vi "tankdataOLD.vi"(7 "LabVIEW Web Service Request":refnum<class "Web Request.lvclass">) -> ()   [LabVIEW 2019]
uses:
  <vilib>/wsapi/Web Request.lvclass
  Type Defs/JSON_Channel.ctl
  Type Defs/JSON_Pump.ctl
panel:
  # "Use the Web Service Request input terminal to call the VIs on the Web Services palette. Do not remove it from the connector pane unless you don't need access to the palette."
  # "Each additional control wired to the connector pane will be available as an input in the URL. To include an indicator in terminal-mode output (the default setting), it must also be wired to the connector pane."
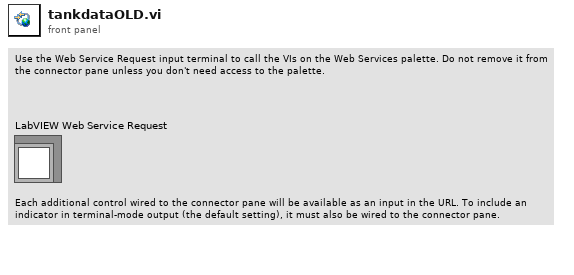
[diagram p1: front panel]
types:
  T1 = typedef "JSON_Tank.ctl" = cluster{"number":u16, "building":string, "room":string, "ipAddress":string, "profileName":string, "caNumber":string, "ctrlType":string, "mode":string, "channels":T2[], "pumps":T3[]}
  T2 = typedef "JSON_Channel.ctl" = cluster{"name":string, "tag":string, "data":string, "type":string, "unit":string}
  T3 = typedef "JSON_Pump.ctl" = cluster{"position":u8, "enabled":bool, "command":string, "channels":T2[], "elapsedTime":string}
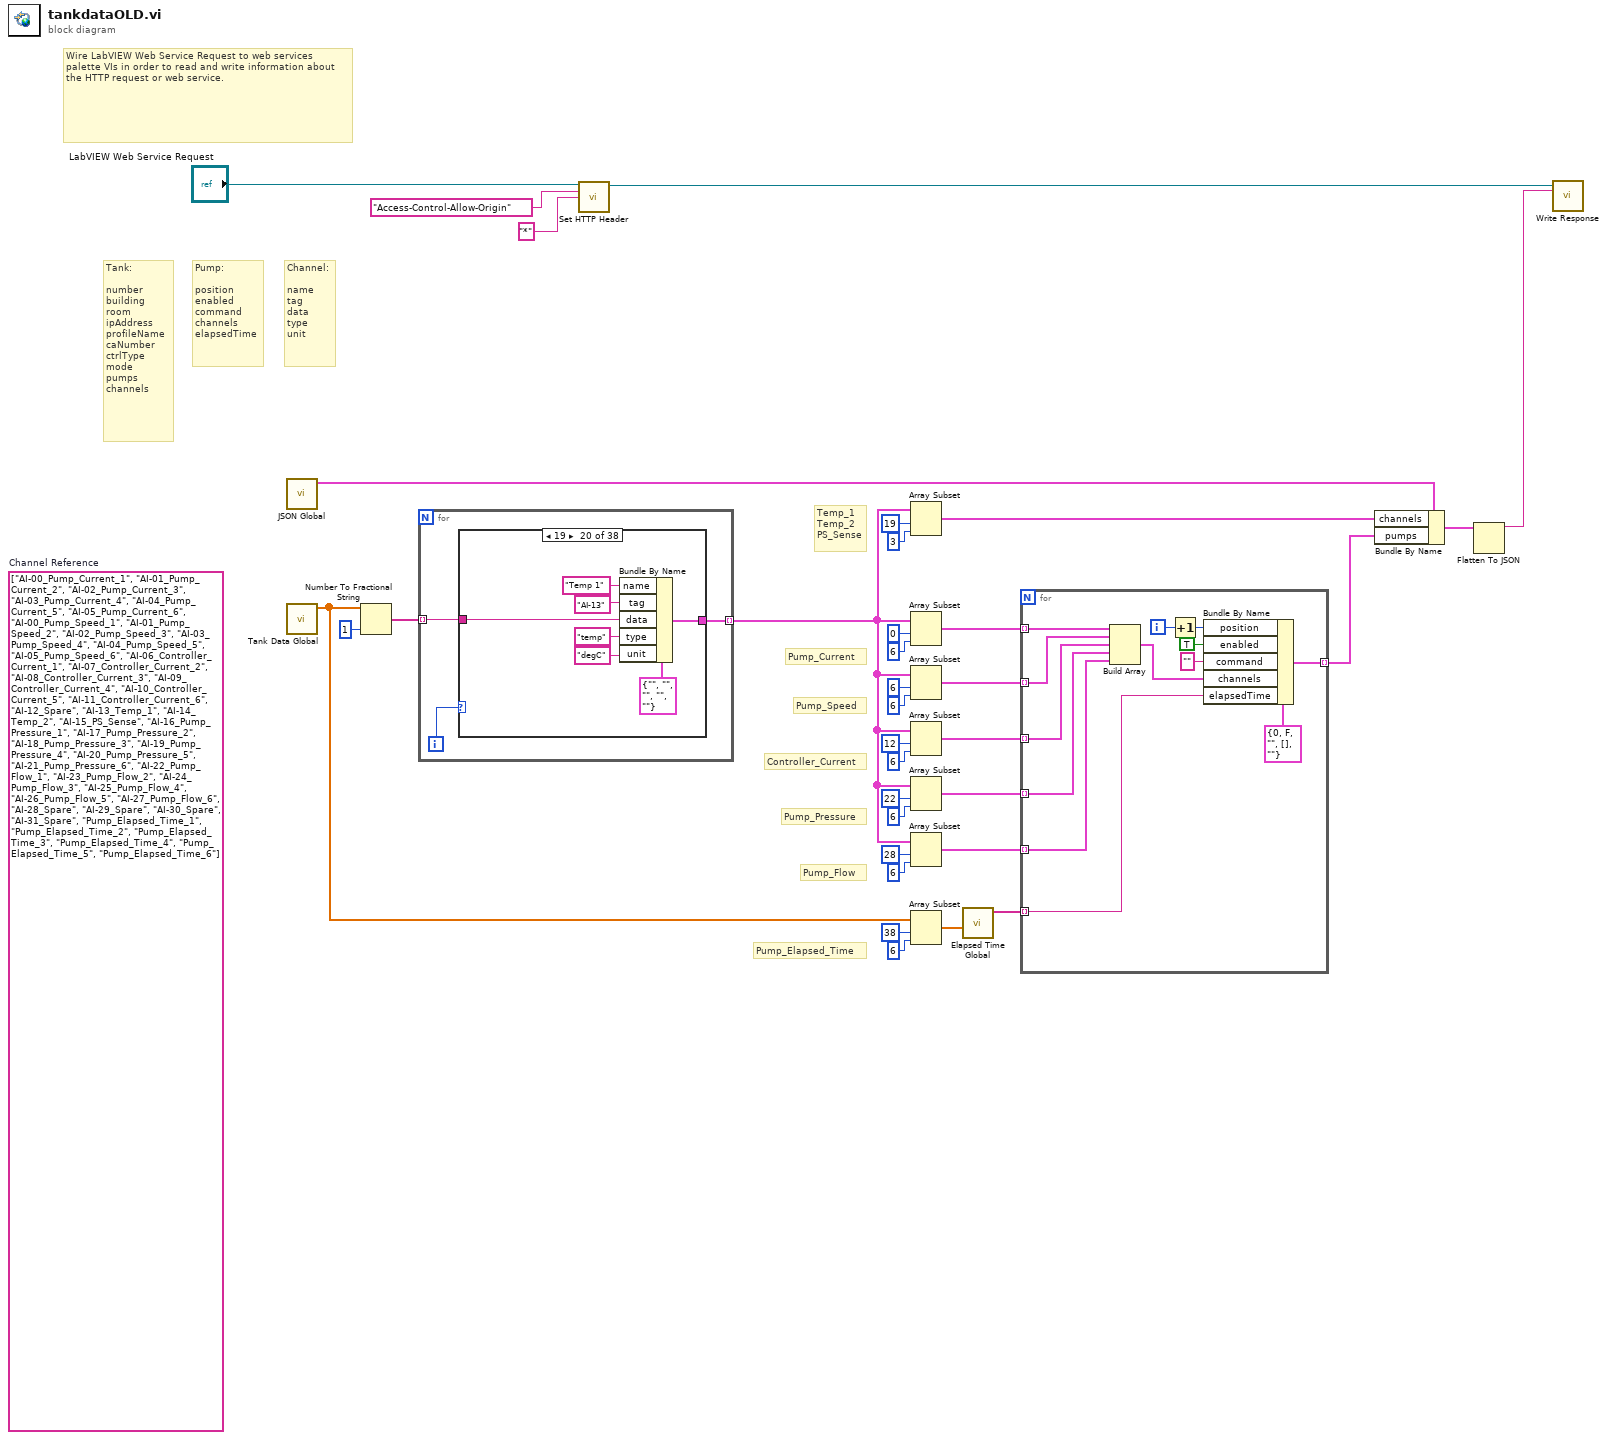
[diagram p0: block diagram]
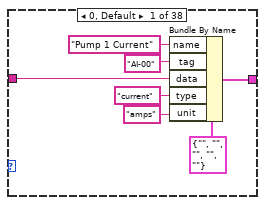
[diagram p2: hidden frame]
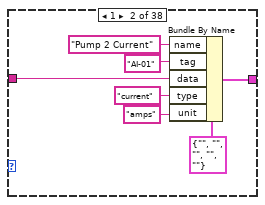
[diagram p3: hidden frame]
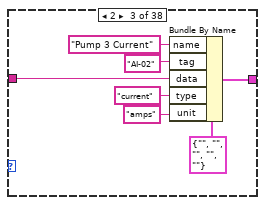
[diagram p4: hidden frame]
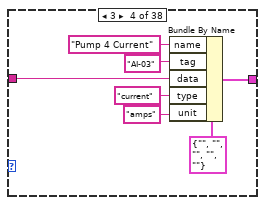
[diagram p5: hidden frame]
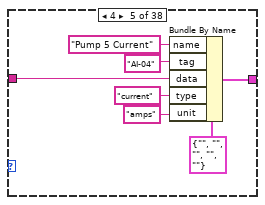
[diagram p6: hidden frame]
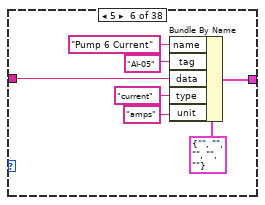
[diagram p7: hidden frame]
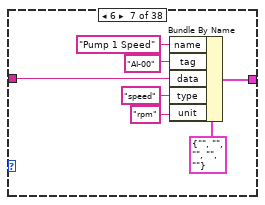
[diagram p8: hidden frame]
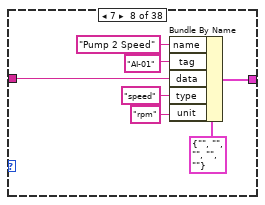
[diagram p9: hidden frame]
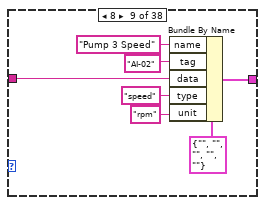
[diagram p10: hidden frame]
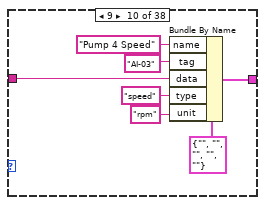
[diagram p11: hidden frame]
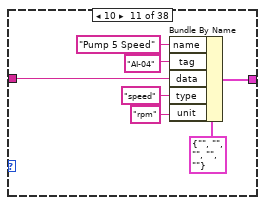
[diagram p12: hidden frame]
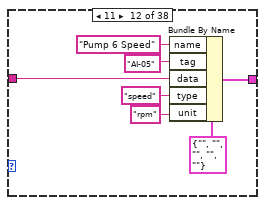
[diagram p13: hidden frame]
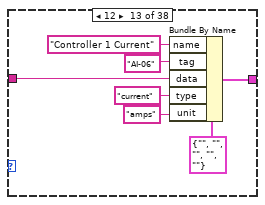
[diagram p14: hidden frame]
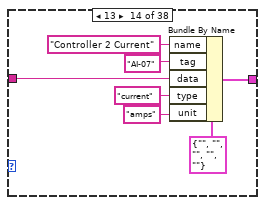
[diagram p15: hidden frame]
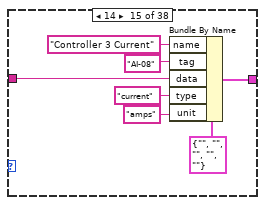
[diagram p16: hidden frame]
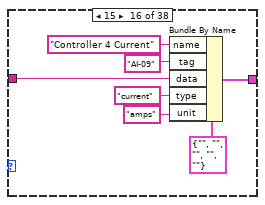
[diagram p17: hidden frame]
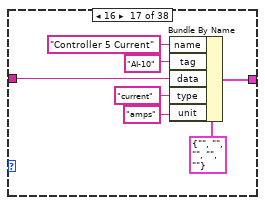
[diagram p18: hidden frame]
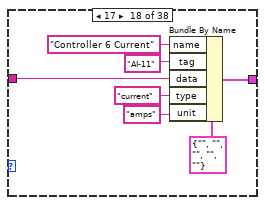
[diagram p19: hidden frame]
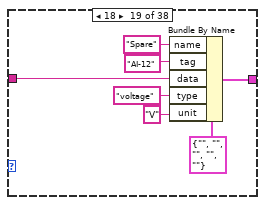
[diagram p20: hidden frame]
diagram:
  (unwired) string[] ["AI-00_Pump_Current_1", "AI-01_Pump_Current_2", "AI-02_Pump_Current_3", "AI-03_Pump_Current_4", "AI-04_Pump_Current_5", "AI-05_Pump_Current_6", "AI-00_Pump_Speed_1", "AI-01_Pump_Speed_2", "AI-02_Pump_Speed_3", "AI-03_Pump_Speed_4", "AI-04_Pump_Speed_5", "AI-05_Pump_Speed_6", "AI-06_Controller_Current_1", "AI-07_Controller_Current_2", "AI-08_Controller_Current_3", "AI-09_Controller_Current_4", "AI-10_Controller_Current_5", "AI-11_Controller_Current_6", "AI-12_Spare", "AI-13_Temp_1", "AI-14_Temp_2", "AI-15_PS_Sense", "AI-16_Pump_Pressure_1", "AI-17_Pump_Pressure_2", "AI-18_Pump_Pressure_3", "AI-19_Pump_Pressure_4", "AI-20_Pump_Pressure_5", "AI-21_Pump_Pressure_6", "AI-22_Pump_Flow_1", "AI-23_Pump_Flow_2", "AI-24_Pump_Flow_3", "AI-25_Pump_Flow_4", "AI-26_Pump_Flow_5", "AI-27_Pump_Flow_6", "AI-28_Spare", "AI-29_Spare", "AI-30_Spare", "AI-31_Spare", "Pump_Elapsed_Time_1", "Pump_Elapsed_Time_2", "Pump_Elapsed_Time_3", "Pump_Elapsed_Time_4", "Pump_Elapsed_Time_5", "Pump_Elapsed_Time_6"]  # Channel Reference
  # "Temp_1\nTemp_2\nPS_Sense"
  # "Pump_Elapsed_Time"
  # "Pump_Flow"
  # "Pump_Pressure"
  # "Controller_Current"
  # "Pump_Speed"
  # "Pump_Current"
  # "Tank:\n\nnumber\nbuilding\nroom\nipAddress\nprofileName\ncaNumber\nctrlType\nmode\npumps\nchannels"
  # "Channel:\n\nname\ntag\ndata\ntype\nunit"
  # "Pump:\n\nposition\nenabled\ncommand\nchannels\nelapsedTime"
  # "Wire LabVIEW Web Service Request to web services palette VIs in order to read and write information about the HTTP request or web service."
  n1 = call "JSON Global.vi"() -> ("JSON Out"=w9:T1)  [unwired: 11 in]
  n2 = call "Tank Data Global.vi"() -> ("Tank Data OUT"=w11:dbl[])  [unwired: 11 in]
  n3 = Number To Fractional String(number=w11, precision (6)=i16 1) -> (F-format string=w17:string[])  [unwired: 2 in]
  n4 = for {
    tunnel: w17 -> [w36] mode=indexing
    tunnel: [w35] -> w6 mode=indexing
    i -> [w37]
    n5 = case shown="19" w37 {
      tunnel: w36 -> [w44 w51 w58 w65 w72 w79 w86 w93 w100 w107 w114 w121 w128 w135 w142 w149 w156 w163 w170 w177 w184 w191 w198 w205 w212 w219 w226 w233 w240 w247 w254 w261 w268 w275 w282 w289 w296 w303]
      tunnel: [w42 w49 w56 w63 w70 w77 w84 w91 w98 w105 w112 w119 w126 w133 w140 w147 w154 w161 w168 w175 w182 w189 w196 w203 w210 w217 w224 w231 w238 w245 w252 w259 w266 w273 w280 w287 w294 w301] -> w35
      frame 0, Default {
        n6 = Bundle By Name(cluster=T2 {"name"="", "tag"="", "data"="", "type"="", "unit"=""} ("Cluster"), "name"="Pump 1 Current", "tag"="AI-00" ("name"), "data"=w44, "type"="current", "unit"="amps") -> (w42:T2)
      }
      frame 1 {
        n7 = Bundle By Name(cluster=T2 {"name"="", "tag"="", "data"="", "type"="", "unit"=""} ("Cluster"), "name"="Pump 2 Current", "tag"="AI-01" ("name"), "data"=w51, "type"="current", "unit"="amps") -> (w49:T2)
      }
      frame 2 {
        n8 = Bundle By Name(cluster=T2 {"name"="", "tag"="", "data"="", "type"="", "unit"=""} ("Cluster"), "name"="Pump 3 Current", "tag"="AI-02" ("name"), "data"=w58, "type"="current", "unit"="amps") -> (w56:T2)
      }
      frame 3 {
        n9 = Bundle By Name(cluster=T2 {"name"="", "tag"="", "data"="", "type"="", "unit"=""} ("Cluster"), "name"="Pump 4 Current", "tag"="AI-03" ("name"), "data"=w65, "type"="current", "unit"="amps") -> (w63:T2)
      }
      frame 4 {
        n10 = Bundle By Name(cluster=T2 {"name"="", "tag"="", "data"="", "type"="", "unit"=""} ("Cluster"), "name"="Pump 5 Current", "tag"="AI-04" ("name"), "data"=w72, "type"="current", "unit"="amps") -> (w70:T2)
      }
      frame 5 {
        n11 = Bundle By Name(cluster=T2 {"name"="", "tag"="", "data"="", "type"="", "unit"=""} ("Cluster"), "name"="Pump 6 Current", "tag"="AI-05" ("name"), "data"=w79, "type"="current", "unit"="amps") -> (w77:T2)
      }
      frame 6 {
        n12 = Bundle By Name(cluster=T2 {"name"="", "tag"="", "data"="", "type"="", "unit"=""} ("Cluster"), "name"="Pump 1 Speed", "tag"="AI-00" ("name"), "data"=w86, "type"="speed", "unit"="rpm") -> (w84:T2)
      }
      frame 7 {
        n13 = Bundle By Name(cluster=T2 {"name"="", "tag"="", "data"="", "type"="", "unit"=""} ("Cluster"), "name"="Pump 2 Speed", "tag"="AI-01" ("name"), "data"=w93, "type"="speed", "unit"="rpm") -> (w91:T2)
      }
      frame 8 {
        n14 = Bundle By Name(cluster=T2 {"name"="", "tag"="", "data"="", "type"="", "unit"=""} ("Cluster"), "name"="Pump 3 Speed", "tag"="AI-02" ("name"), "data"=w100, "type"="speed", "unit"="rpm") -> (w98:T2)
      }
      frame 9 {
        n15 = Bundle By Name(cluster=T2 {"name"="", "tag"="", "data"="", "type"="", "unit"=""} ("Cluster"), "name"="Pump 4 Speed", "tag"="AI-03" ("name"), "data"=w107, "type"="speed", "unit"="rpm") -> (w105:T2)
      }
      frame 10 {
        n16 = Bundle By Name(cluster=T2 {"name"="", "tag"="", "data"="", "type"="", "unit"=""} ("Cluster"), "name"="Pump 5 Speed", "tag"="AI-04" ("name"), "data"=w114, "type"="speed", "unit"="rpm") -> (w112:T2)
      }
      frame 11 {
        n17 = Bundle By Name(cluster=T2 {"name"="", "tag"="", "data"="", "type"="", "unit"=""} ("Cluster"), "name"="Pump 6 Speed", "tag"="AI-05" ("name"), "data"=w121, "type"="speed", "unit"="rpm") -> (w119:T2)
      }
      frame 12 {
        n18 = Bundle By Name(cluster=T2 {"name"="", "tag"="", "data"="", "type"="", "unit"=""} ("Cluster"), "name"="Controller 1 Current", "tag"="AI-06" ("name"), "data"=w128, "type"="current", "unit"="amps") -> (w126:T2)
      }
      frame 13 {
        n19 = Bundle By Name(cluster=T2 {"name"="", "tag"="", "data"="", "type"="", "unit"=""} ("Cluster"), "name"="Controller 2 Current", "tag"="AI-07" ("name"), "data"=w135, "type"="current", "unit"="amps") -> (w133:T2)
      }
      frame 14 {
        n20 = Bundle By Name(cluster=T2 {"name"="", "tag"="", "data"="", "type"="", "unit"=""} ("Cluster"), "name"="Controller 3 Current", "tag"="AI-08" ("name"), "data"=w142, "type"="current", "unit"="amps") -> (w140:T2)
      }
      frame 15 {
        n21 = Bundle By Name(cluster=T2 {"name"="", "tag"="", "data"="", "type"="", "unit"=""} ("Cluster"), "name"="Controller 4 Current", "tag"="AI-09" ("name"), "data"=w149, "type"="current", "unit"="amps") -> (w147:T2)
      }
      frame 16 {
        n22 = Bundle By Name(cluster=T2 {"name"="", "tag"="", "data"="", "type"="", "unit"=""} ("Cluster"), "name"="Controller 5 Current", "tag"="AI-10" ("name"), "data"=w156, "type"="current", "unit"="amps") -> (w154:T2)
      }
      frame 17 {
        n23 = Bundle By Name(cluster=T2 {"name"="", "tag"="", "data"="", "type"="", "unit"=""} ("Cluster"), "name"="Controller 6 Current", "tag"="AI-11" ("name"), "data"=w163, "type"="current", "unit"="amps") -> (w161:T2)
      }
      frame 18 {
        n24 = Bundle By Name(cluster=T2 {"name"="", "tag"="", "data"="", "type"="", "unit"=""} ("Cluster"), "name"="Spare", "tag"="AI-12" ("name"), "data"=w170, "type"="voltage", "unit"="V") -> (w168:T2)
      }
      frame 19 {
        n25 = Bundle By Name(cluster=T2 {"name"="", "tag"="", "data"="", "type"="", "unit"=""} ("Cluster"), "name"="Temp 1", "tag"="AI-13" ("name"), "data"=w177, "type"="temp", "unit"="degC") -> (w175:T2)
      }
      frame 20 {
        n26 = Bundle By Name(cluster=T2 {"name"="", "tag"="", "data"="", "type"="", "unit"=""} ("Cluster"), "name"="Temp 2", "tag"="AI-14" ("name"), "data"=w184, "type"="temp", "unit"="degC") -> (w182:T2)
      }
      frame 21 {
        n27 = Bundle By Name(cluster=T2 {"name"="", "tag"="", "data"="", "type"="", "unit"=""} ("Cluster"), "name"="PS Sense", "tag"="AI-15" ("name"), "data"=w191, "type"="voltage", "unit"="V") -> (w189:T2)
      }
      frame 22 {
        n28 = Bundle By Name(cluster=T2 {"name"="", "tag"="", "data"="", "type"="", "unit"=""} ("Cluster"), "name"="Pump 1 Pressure", "tag"="AI-16" ("name"), "data"=w198, "type"="pressure", "unit"="kPa") -> (w196:T2)
      }
      frame 23 {
        n29 = Bundle By Name(cluster=T2 {"name"="", "tag"="", "data"="", "type"="", "unit"=""} ("Cluster"), "name"="Pump 2 Pressure", "tag"="AI-17" ("name"), "data"=w205, "type"="pressure", "unit"="kPa") -> (w203:T2)
      }
      frame 24 {
        n30 = Bundle By Name(cluster=T2 {"name"="", "tag"="", "data"="", "type"="", "unit"=""} ("Cluster"), "name"="Pump 3 Pressure", "tag"="AI-18" ("name"), "data"=w212, "type"="pressure", "unit"="kPa") -> (w210:T2)
      }
      frame 25 {
        n31 = Bundle By Name(cluster=T2 {"name"="", "tag"="", "data"="", "type"="", "unit"=""} ("Cluster"), "name"="Pump 4 Pressure", "tag"="AI-19" ("name"), "data"=w219, "type"="pressure", "unit"="kPa") -> (w217:T2)
      }
      frame 26 {
        n32 = Bundle By Name(cluster=T2 {"name"="", "tag"="", "data"="", "type"="", "unit"=""} ("Cluster"), "name"="Pump 5 Pressure", "tag"="AI-20" ("name"), "data"=w226, "type"="pressure", "unit"="kPa") -> (w224:T2)
      }
      frame 27 {
        n33 = Bundle By Name(cluster=T2 {"name"="", "tag"="", "data"="", "type"="", "unit"=""} ("Cluster"), "name"="Pump 6 Pressure", "tag"="AI-21" ("name"), "data"=w233, "type"="pressure", "unit"="kPa") -> (w231:T2)
      }
      frame 28 {
        n34 = Bundle By Name(cluster=T2 {"name"="", "tag"="", "data"="", "type"="", "unit"=""} ("Cluster"), "name"="Pump 1 Flow", "tag"="AI-22" ("name"), "data"=w240, "type"="flow", "unit"="lph") -> (w238:T2)
      }
      frame 29 {
        n35 = Bundle By Name(cluster=T2 {"name"="", "tag"="", "data"="", "type"="", "unit"=""} ("Cluster"), "name"="Pump 2 Flow", "tag"="AI-23" ("name"), "data"=w247, "type"="flow", "unit"="lph") -> (w245:T2)
      }
      frame 30 {
        n36 = Bundle By Name(cluster=T2 {"name"="", "tag"="", "data"="", "type"="", "unit"=""} ("Cluster"), "name"="Pump 3 Flow", "tag"="AI-24" ("name"), "data"=w254, "type"="flow", "unit"="lph") -> (w252:T2)
      }
      frame 31 {
        n37 = Bundle By Name(cluster=T2 {"name"="", "tag"="", "data"="", "type"="", "unit"=""} ("Cluster"), "name"="Pump 4 Flow", "tag"="AI-25" ("name"), "data"=w261, "type"="flow", "unit"="lph") -> (w259:T2)
      }
      frame 32 {
        n38 = Bundle By Name(cluster=T2 {"name"="", "tag"="", "data"="", "type"="", "unit"=""} ("Cluster"), "name"="Pump 5 Flow", "tag"="AI-26" ("name"), "data"=w268, "type"="flow", "unit"="lph") -> (w266:T2)
      }
      frame 33 {
        n39 = Bundle By Name(cluster=T2 {"name"="", "tag"="", "data"="", "type"="", "unit"=""} ("Cluster"), "name"="Pump 6 Flow", "tag"="AI-27" ("name"), "data"=w275, "type"="flow", "unit"="lph") -> (w273:T2)
      }
      frame 34 {
        n40 = Bundle By Name(cluster=T2 {"name"="", "tag"="", "data"="", "type"="", "unit"=""} ("Cluster"), "name"="Spare", "tag"="AI-28" ("name"), "data"=w282, "type"="voltage", "unit"="V") -> (w280:T2)
      }
      frame 35 {
        n41 = Bundle By Name(cluster=T2 {"name"="", "tag"="", "data"="", "type"="", "unit"=""} ("Cluster"), "name"="Spare", "tag"="AI-29" ("name"), "data"=w289, "type"="voltage", "unit"="V") -> (w287:T2)
      }
      frame 36 {
        n42 = Bundle By Name(cluster=T2 {"name"="", "tag"="", "data"="", "type"="", "unit"=""} ("Cluster"), "name"="Spare", "tag"="AI-30" ("name"), "data"=w296, "type"="voltage", "unit"="V") -> (w294:T2)
      }
      frame 37 {
        n43 = Bundle By Name(cluster=T2 {"name"="", "tag"="", "data"="", "type"="", "unit"=""} ("Cluster"), "name"="Spare", "tag"="AI-31" ("name"), "data"=w303, "type"="voltage", "unit"="V") -> (w301:T2)
      }
    }
  }
  n44 = call <vilib>:"Set HTTP Header.vi"("LabVIEW Web Service Request"="LabVIEW Web Service Request", "header"="Access-Control-Allow-Origin" ("header value"), "header value"="*" ("header")) -> ("LabVIEW Web Service Request out"=w33:refnum<class "Web Request.lvclass">)  [unwired: 11 in, 1 out]
  n45 = Array Subset(array=w6, index=19, length=3 ("index")) -> (w5:T2[])
  n46 = Array Subset(array=w6, index=0, length=6 ("index")) -> (w16:T2[])
  n47 = Array Subset(array=w6, index=6, length=6 ("index")) -> (w15:T2[])
  n48 = Array Subset(array=w6, index=12, length=6 ("index")) -> (w14:T2[])
  n49 = Array Subset(array=w6, index=22, length=6 ("index")) -> (w13:T2[])
  n50 = Array Subset(array=w6, index=28, length=6 ("index")) -> (w12:T2[])
  n51 = Array Subset(array=w11, index=38, length=6 ("index")) -> (w10:dbl[])
  n52 = call "Elapsed Time Global.vi"("Ticks IN"=w10) -> ("Elapsed Times"=w1:string[])  [unwired: 10 in]
  n53 = for {
    tunnel: w16 -> [w316] mode=indexing
    tunnel: w15 -> [w315] mode=indexing
    tunnel: w14 -> [w314] mode=indexing
    tunnel: w13 -> [w313] mode=indexing
    tunnel: w12 -> [w312] mode=indexing
    tunnel: w1 -> [w306] mode=indexing
    tunnel: [w305] -> w4 mode=indexing
    i -> [w310]
    n54 = Build Array(w316, w315, w314, w313, w312) -> (w307:T2[])
    n55 = Increment(x=w310) -> (x+1=w304:i32)
    n56 = Bundle By Name(cluster=T3 {"position"=0, "enabled"=FALSE, "command"="", "channels"=[], "elapsedTime"=""}, "position"=w304, "enabled"=TRUE, "command"="", "channels"=w307, "elapsedTime"=w306) -> (w305:T3)
  }
  n57 = Bundle By Name(cluster=w9, "channels"=w5, "pumps"=w4) -> (w3:T1)
  n58 = Flatten To JSON(anything=w3) -> (JSON string=w2:string)  [unwired: 2 in, 1 out]
  n59 = call <vilib>:"Write Response.vi"("LabVIEW Web Service Request"=w33, "response string"=w2) -> ()  [unwired: 12 in, 2 out]
